vi "Command v1.3.vi"() -> ()   [LabVIEW 2019]
uses:
  <vilib>/ptbypt/NI_PtbyPt.lvlib
panel:
  in  "FU BUTTON FEEDBACK":dbl[](array[numeric])
  out "Array - Numeric":dbl[](array[numeric])
  out "PH LED 6":bool=TRUE
  in  "PH CHECK 6":bool
  out "PH IND 6":bool=TRUE
  in  "CYCLE OX VENT BUTTON":bool
  in  "CYCLE FUEL VENT BUTTON":bool
  in  "DATA INPUT":dbl[](array[numeric])
  in  "INDICATOR INPUT":dbl[](array[numeric])
  out "PH LED 5":bool=TRUE
  out "PH LED 4":bool=TRUE
  out "PH LED 3":bool=TRUE
  out "PH LED 2":bool=TRUE
  out "PH LED 1":bool=TRUE
  in  "PH CHECK 1":bool
  in  "PH CHECK 2":bool
  in  "PH CHECK 3":bool
  in  "PH CHECK 4":bool
  in  "PH CHECK 5":bool
  out "PH IND 5":bool=TRUE
  out "PH IND 4":bool=TRUE
  out "PH IND 3":bool=TRUE
  out "PH IND 2":bool=TRUE
  out "PH IND 1":bool=TRUE
  out "IGN INSERTED BUTTON LED":bool
  in  "IGNITOR IN BUTTON":bool
  in  "MISC BUTTON":bool
  in  "WATER SUP BUTTON":bool
  out "ENGINE TEMP GNG":bool=TRUE
  out "ENGINE PRESS GNG":bool=TRUE
  out "IGNITOR GNG":bool=TRUE
  out "STARTUP GNG":bool=TRUE
  out "SUB PANELS GNG":bool=TRUE
  out "SUB PANEL OX GNG NUM":dbl
  out "SUB PANEL OX GNG LED":bool=TRUE
  out "SUB PANEL FU GNG NUM":dbl
  out "SUB PANEL FU GNG LED":bool=TRUE
  out "VALVE STATES GNG":bool=TRUE
  out "VAVLES ST OX GNG NUM":dbl
  out "VALVE ST OX GNG LED":bool=TRUE
  out "VALVE ST FU GNG NUM":dbl
  out "VALVE ST FU GNG LED":bool=TRUE
  out "PURGE GNG":bool=TRUE
  out "PURGE GNG NUM":dbl
  out "PURGE GNG LED":bool=TRUE
  out "WATER SUP GNG":bool=TRUE
  out "WATER SUP GNG NUM":dbl
  out "WATER SUP GNG LED":bool=TRUE
  out "PRESS VALVES GNG":bool=TRUE
  out "PRESS VALVE OX GNG NUM":dbl
  out "PRESS VALVE OX GNG LED":bool=TRUE
  out "PRESS VALVE FU GNG NUM":dbl
  out "PRESS VALVE FU GNG LED":bool=TRUE
  out "OFFICE GNG":bool=TRUE
  out "RECORD GNG":bool=TRUE
  out "OFFICE GNG NUM":dbl
  out "OFFICE GNG LED":bool=TRUE
  out "RECORD GNG NUM":dbl
  out "RECORD GNG LED":bool=TRUE
  in  "DISABLE BUTTON":bool
  in  "PURGE (1 SEC) BUTTON":bool
  in  "PURGE (2 SEC) BUTTON":bool
  out "TANK PRESS OX METER":dbl(knob) scale=0.0..1600.0
  out "REG PRESS OX METER":dbl(knob) scale=0.0..1600.0
  out "TANK PRESS FU METER":dbl(knob) scale=0.0..1600.0
  out "REG PRESS FU METER":dbl(knob) scale=0.0..1600.0
  in  "RESET":bool
  in  "STOP":bool
  out "ARM GNG":bool=TRUE
  out "IGN IN GNG":bool=TRUE
  out "INJ TEMP GNG":bool=TRUE
  out "CAM GNG":bool=TRUE
  out "PRESS BOTTLE GNG":bool=TRUE
  out "CHILL GNG":bool=TRUE
  out "SYS CYCLE GNG":bool=TRUE
  out "FILL VALVES GNG":bool=TRUE
  out "TANK LEVEL GNG":bool=TRUE
  out "VENT CYCLE GNG":bool=TRUE
  out "ISO VALVE GNG":bool=TRUE
  out "TANK PRESS GNG":bool=TRUE
  out "REG PRESS GNG":bool=TRUE
  out "RELIEF GNG":bool=TRUE
  out "NANNY GNG":bool=TRUE
  out "INJ TEMP GNG NUM":dbl
  out "INJ TEMP GNG LED":bool=TRUE
  out "FILL VALVE OX GNG NUM":dbl
  out "FILL VALVE OX GNG LED":bool=TRUE
  out "ARMED GNG NUM":dbl
  out "ARMED GNG LED":bool=TRUE
  out "TANK LEVEL OX GNG NUM":dbl
  out "TANK LEVEL OX GNG LED":bool=TRUE
  out "VENT CYCLE OX GNG NUM":dbl
  out "VENT CYCLE OX GNG LED":bool=TRUE
  out "PRESS BOTTLE GNG NUM":dbl
  out "PRESS BOTTLE GNG LED":bool=TRUE
  out "ISO VALVE OX GNG NUM":dbl
  out "ISO VALVE OX GNG LED":bool=TRUE
  out "TANK PRESS OX GNG NUM":dbl
  out "TANK PRESS OX GNG LED":bool=TRUE
  out "REG PRESS OX GNG NUM":dbl
  out "REG PRESS OX GNG LED":bool=TRUE
  out "RELIEF OX GNG NUM":dbl
  out "RELIEF OX GNG LED":bool=TRUE
  out "VALVE CYCLE GNG NUM":dbl
  out "SYS CYCLE GNG LED":bool=TRUE
  out "CAM GNG NUM":dbl
  out "CAM GNG LED":bool=TRUE
  out "IGN IN GNG NUM":dbl
  out "IGN IN GNG LED":bool=TRUE
  out "FILL VALVE FU GNG NUM":dbl
  out "FILL VALVE FU GNG LED":bool=TRUE
  out "TANK LEVEL FU GNG NUM":dbl
  out "TANK LEVEL FU GNG LED":bool=TRUE
  out "VENT CYCLE FU GNG NUM":dbl
  out "VENT CYCLE FU GNG LED":bool=TRUE
  out "CHILL GNG NUM":dbl
  out "CHILL GNG LED":bool=TRUE
  out "ISO VALVE FU GNG NUM":dbl
  out "ISO VALVE FU GNG LED":bool=TRUE
  out "TANK PRESS FU GNG NUM":dbl
  out "TANK PRESS FU GNG LED":bool=TRUE
  out "REG PRESS FU GNG NUM":dbl
  out "REG PRESS FU GNG LED":bool=TRUE
  out "RELIEF FU GNG NUM":dbl
  out "RELIEF FU GNG LED":bool=TRUE
  out "NANNY GNG NUM":dbl
  out "NANNY GNG LED":bool=TRUE
  in  "STARTUP BUTTON":bool
  out "PT COMBUSTION CHAMBER":dbl
  in  "SYS GNG BUTTON":bool=TRUE
  out "REC DATA BUTTON LED":bool
  in  "RECORD DATA BUTTON":bool
  out "CC TEMP 3":dbl(slide) scale=-150.0..500.0
  out "CC TEMP 2":dbl(slide) scale=-150.0..500.0
  out "CC TEMP 1":dbl(slide) scale=-150.0..500.0
  out "OX CHILL TEMP":dbl(slide) scale=-200.0..75.0
  out "OFFICE GNG BUTTON LED":bool
  in  "OFFICE GNG BUTTON":bool
  out "CAM GNG BUTTON LED":bool
  in  "CAM GNG BUTTON":bool
  out "OX TANK TEMP 4":dbl(slide) scale=-200.0..75.0
  out "OX TANK TEMP 3":dbl(slide) scale=-200.0..75.0
  out "OX TANK TEMP 5":dbl(slide) scale=-200.0..75.0
  out "OX TANK TEMP 1":dbl(slide) scale=-200.0..75.0
  out "ARMED PANEL LED":bool
  out "IGN INSERTED PANEL LED":bool
  out "NANNY PAN LED":bool
  out "FUEL VENT CYCLE BUTTON LED":bool
  out "OX VENT CYCLE BUTTON LED":bool
  in  "VALVE SEQ BUTTON":bool
  in  "FIRE BUTTON":bool
  out "PT FU MAIN VALVE":dbl
  out "PT FU VENTURI":dbl
  out "PT OX MAIN VALVE":dbl
  out "PT OX VENTURI":dbl
  out "FUEL TANK RELIEF TEMP":dbl(slide) scale=-200.0..75.0
  out "FUELTANK TEMP":dbl(slide) scale=-200.0..75.0
  out "OX TANK RELIEF TEMP":dbl(slide) scale=-200.0..75.0
  out "OX LINE RELIEF TEMP":dbl(slide) scale=-200.0..75.0
  in  "ABORT BUTTON":bool
  in  "COMMAND GNG BUTTON":bool=TRUE
  out "OX SUB PANEL GNG MAIN":bool=TRUE
  out "FU SUB PANEL GNG MAIN":bool=TRUE
  out "SYS STATE FU STRING":string
  out "SYS STATE OX STRING":string
  out "FUEL TANK LEVEL (%) 2":dbl(slide) scale=0.0..100.0
  in  "ABV-OX-250 (OX FILL)":bool
  out "ABV-OX-250 LED":bool=TRUE
  in  "ABV-OX-240 (OX CHILL)":bool
  out "ABV-OX-240 LED":bool=TRUE
  in  "ABV-OX-230 (OX MAIN)":bool
  out "ABV-OX-230 LED":bool=TRUE
  in  "ABV-OX-220 (OX ISO)":bool
  out "ABV-OX-220 LED":bool=TRUE
  in  "ABV-OX-210 (OX VENT)":bool
  out "ABV-OX-210 LED":bool=TRUE
  in  "ABV-PR-110 (OX PRESS)":bool
  out "ABV-PR-110 LED":bool=TRUE
  in  "NANNY MODE BUTTON":bool
  out "PT PRESSURANT":dbl(slide) scale=0.0..10.0
  out "SYS STATE MAIN STRING":string
  out "FUEL TANK LEVEL (%)":dbl(slide) scale=0.0..100.0
  in  "FUEL FILL BUTTON":bool
  out "FUEL FILL LED":bool=TRUE
  in  "ABV-FU-340 (FUEL PURGE)":bool
  out "ABV-FU-340 LED":bool=TRUE
  in  "ABV-FU-330 (FUEL MAIN)":bool
  out "ABV-FU-330 LED":bool=TRUE
  in  "ABV-FU-320 (FUEL ISO)":bool
  out "ABV-FU-320 LED":bool=TRUE
  in  "ABV-FU-310 (FUEL VENT)":bool
  out "ABV-FU-310 LED":bool=TRUE
  in  "ABV-PR-120 (FUEL PRESS)":bool
  out "ABV-PR-120 LED":bool=TRUE
  # "Ox CONTROL"
  # "FUEL CONTROL"
  # "NANNY"
  # "IGNITOR \nINSERTED"
  # "ARMED"
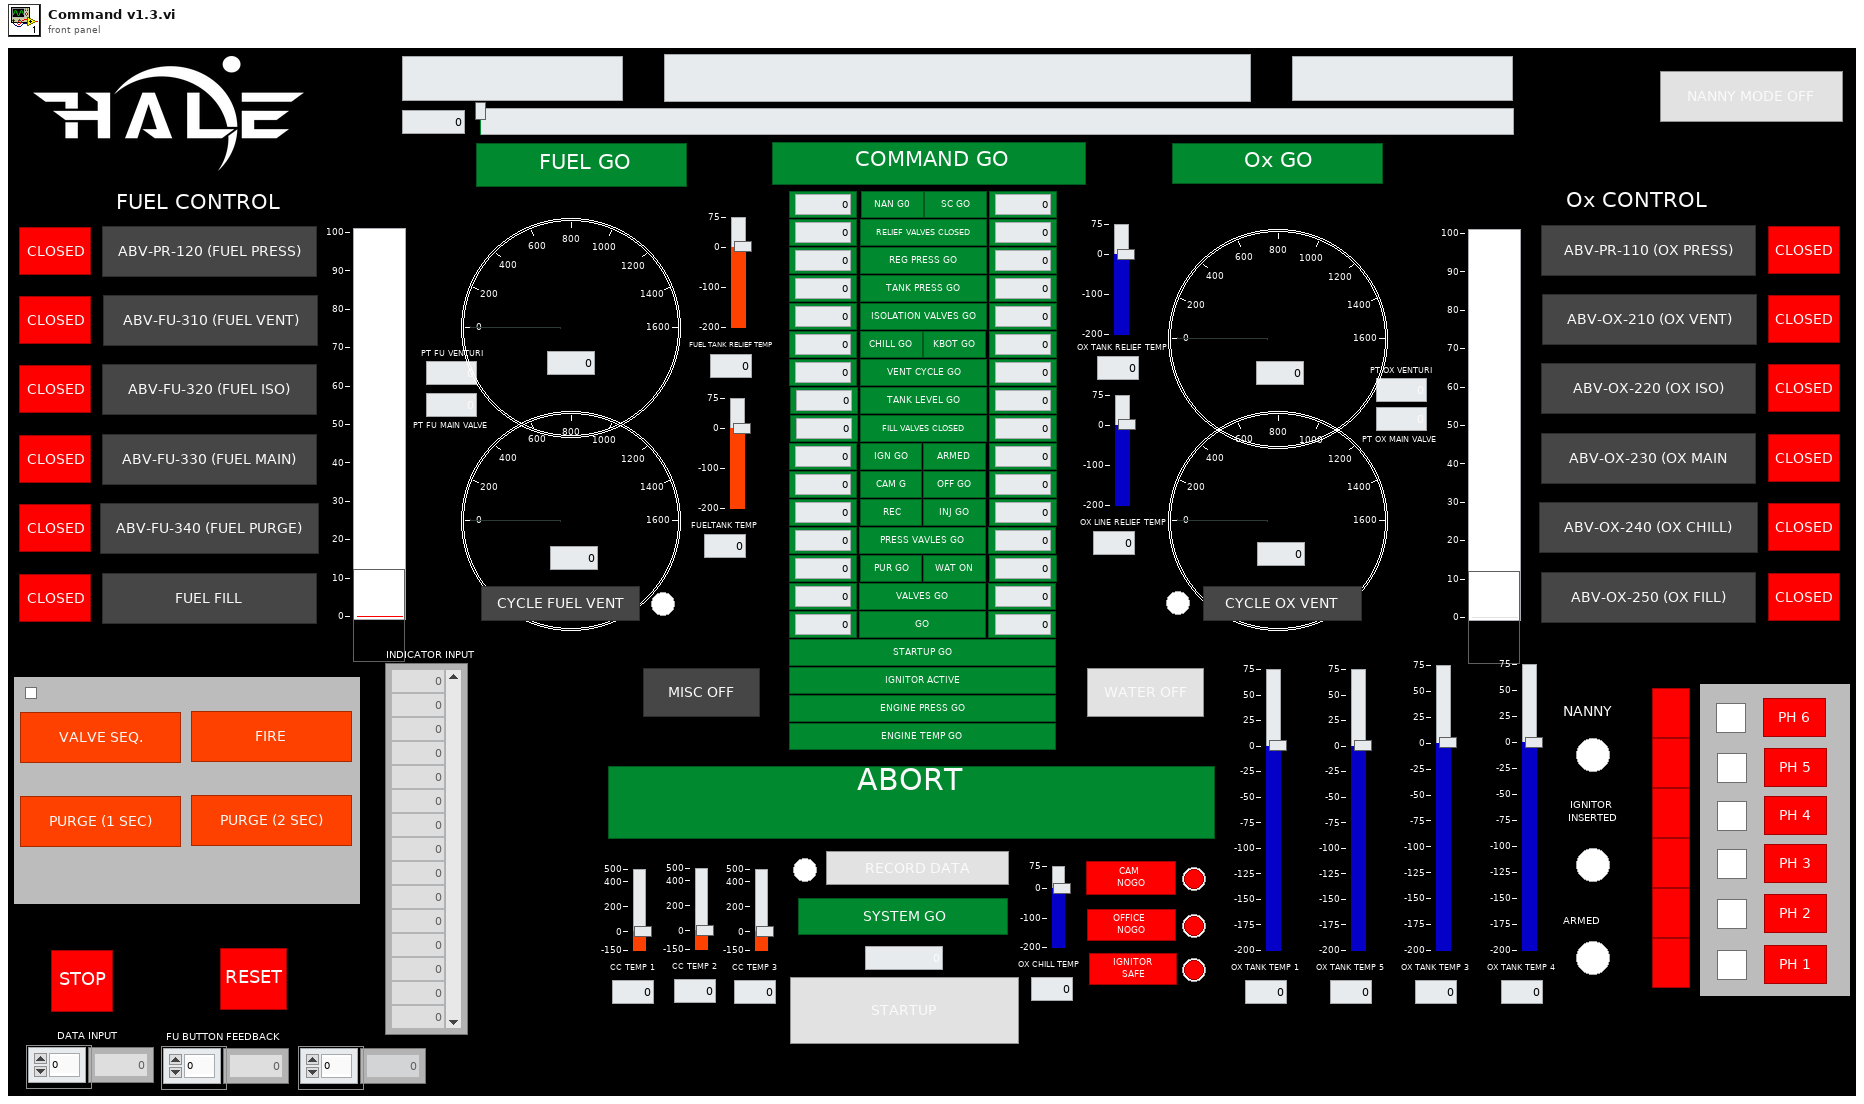
[diagram p1: front panel]
types:
  T1 = enum8{"Enabled", "Disabled", "Disabled and Grayed Out"}
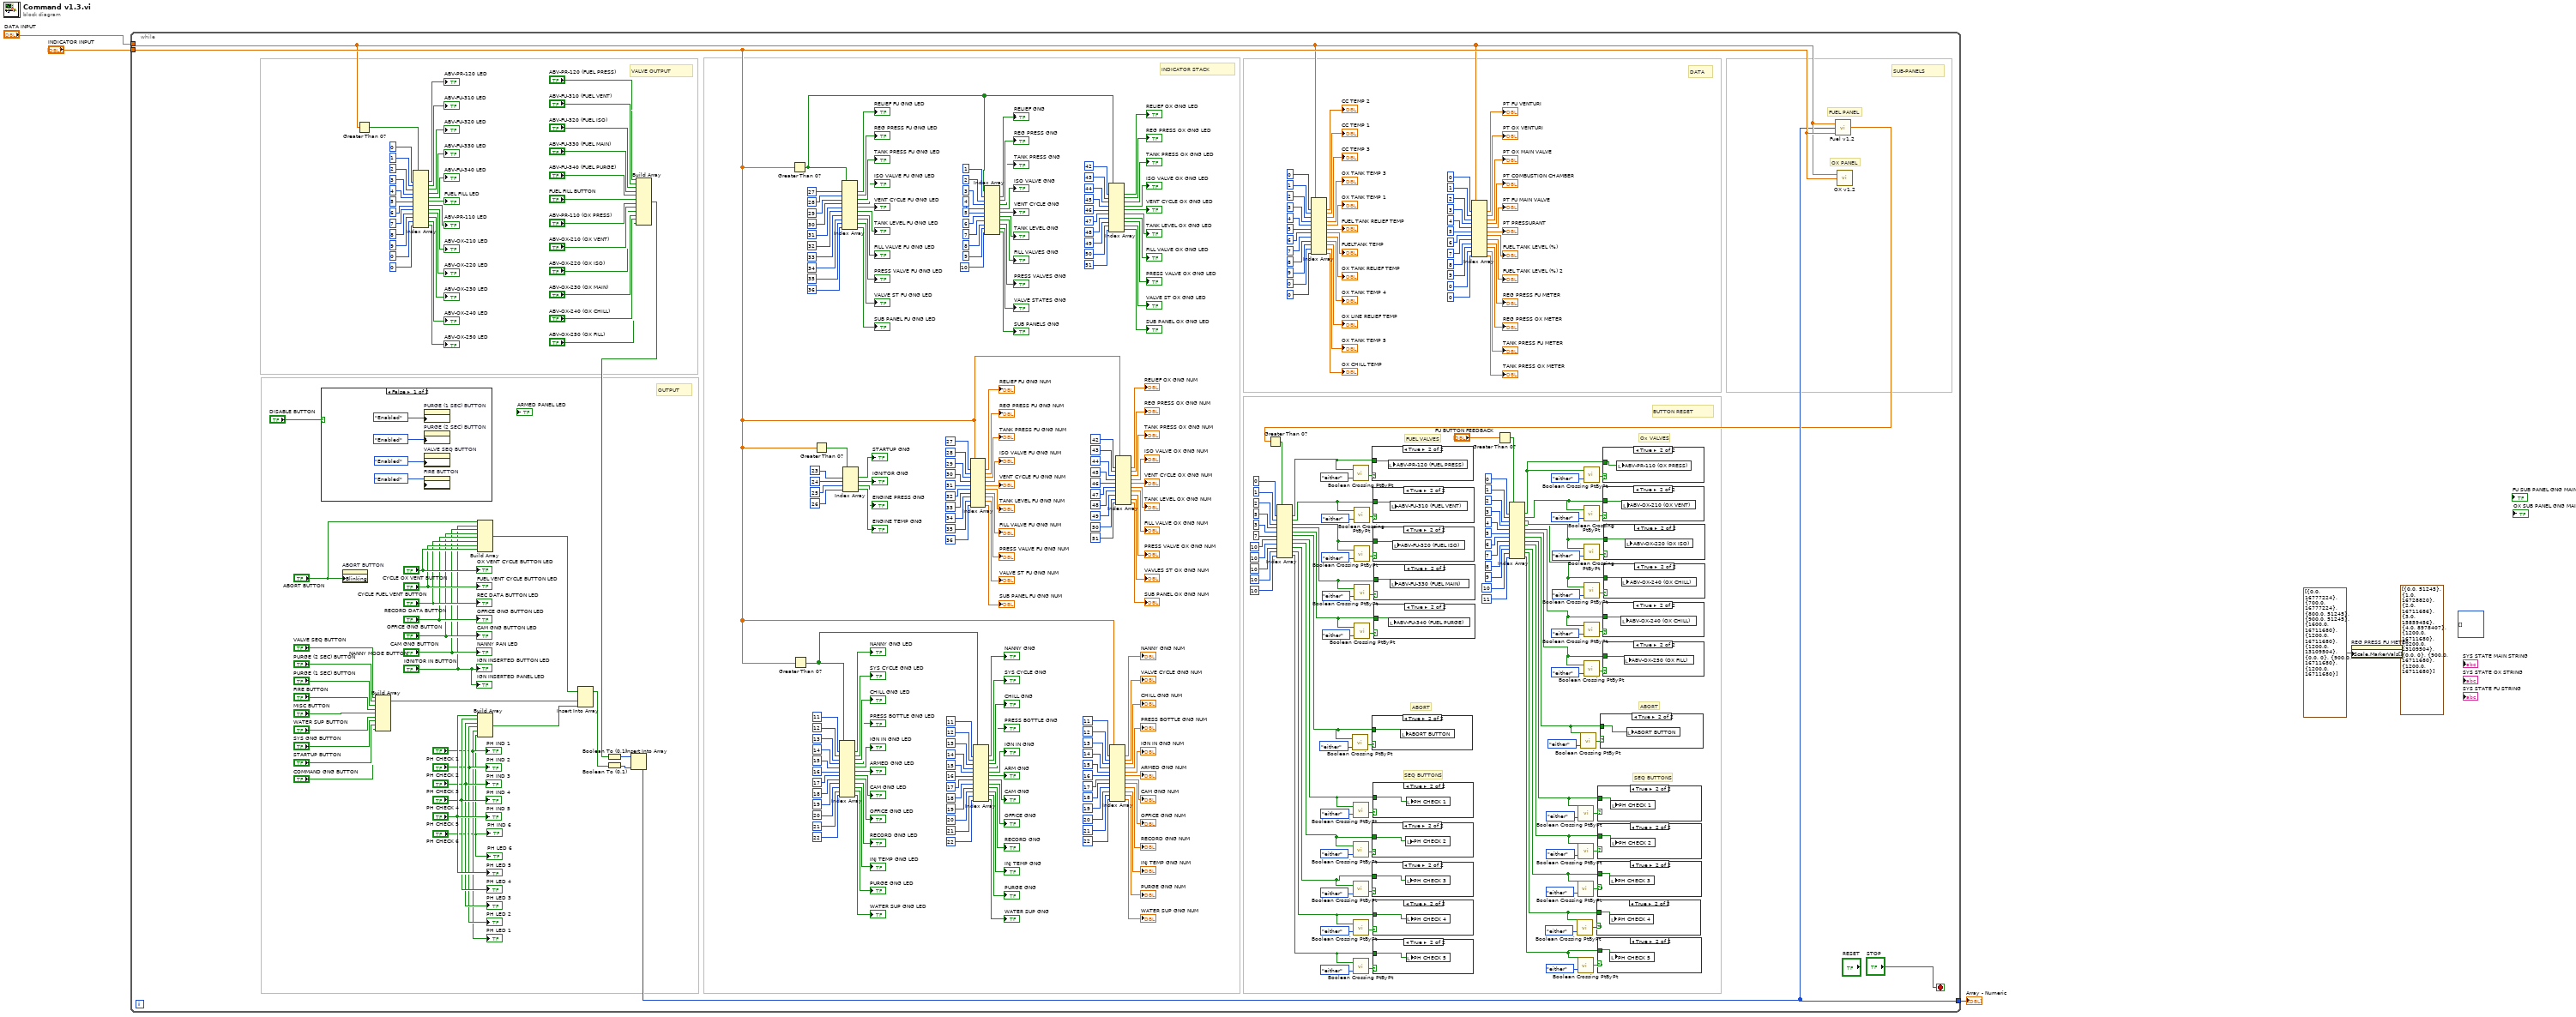
[diagram p0: block diagram]
diagram:
  (unwired) u32[] [] ("Scale.Marker Values[]")
  (unwired) cluster{dbl, u32}[] [{0.0, 51245}, {1.0, 16728820}, {2.0, 16711686}, {3.0, 15859456}, {4.0, 8978407}, {1200.0, 16711680}, {1200.0, 13109504}, {0.0, 0}, {900.0, 16711680}, {1200.0, 16711680}] ("Scale.Marker Values[]")
  n1 = while {
    tunnel: "INDICATOR INPUT" -> [w16]
    tunnel: "DATA INPUT" -> [w15]
    tunnel: [w6] -> w1
    stop <- "STOP" stop-if-true
    # "SUB-PANELS"
    # "FUEL PANEL"
    # "OX PANEL"
    # "SEQ BUTTONS"
    # "ABORT"
    # "SEQ BUTTONS"
    # "ABORT"
    # "FUEL VALVES"
    # "Ox VALVES"
    # "BUTTON RESET"
    # "DATA"
    # "INDICATOR STACK"
    # "VALVE OUTPUT"
    # "OUTPUT"
    n2 = case shown="False" "DISABLE BUTTON" {
      frame False {
        n3 = property on="PURGE (1 SEC) BUTTON" class="Bool (strict)"("DisabledEnum"=T1."Enabled" ("Disabled")) -> ()  [unwired: 2 in, 2 out]
        n4 = property on="PURGE (2 SEC) BUTTON" class="Bool (strict)"("DisabledEnum"=T1."Enabled" ("Disabled")) -> ()  [unwired: 2 in, 2 out]
        n5 = property on="VALVE SEQ BUTTON" class="Bool (strict)"("DisabledEnum"=T1."Enabled" ("Disabled")) -> ()  [unwired: 2 in, 2 out]
        n6 = property on="FIRE BUTTON" class="Bool (strict)"("DisabledEnum"=T1."Enabled" ("Disabled")) -> ()  [unwired: 2 in, 2 out]
      }
      frame True {
        n7 = property on="VALVE SEQ BUTTON" class="Bool (strict)"("DisabledEnum"=T1."Disabled and Grayed Out" ("Disabled")) -> ()  [unwired: 2 in, 2 out]
        n8 = property on="PURGE (2 SEC) BUTTON" class="Bool (strict)"("DisabledEnum"=T1."Disabled and Grayed Out" ("Disabled")) -> ()  [unwired: 2 in, 2 out]
        n9 = property on="FIRE BUTTON" class="Bool (strict)"("DisabledEnum"=T1."Disabled and Grayed Out" ("Disabled")) -> ()  [unwired: 2 in, 2 out]
        n10 = property on="PURGE (1 SEC) BUTTON" class="Bool (strict)"("DisabledEnum"=T1."Disabled and Grayed Out" ("Disabled")) -> ()  [unwired: 2 in, 2 out]
      }
    }
    n11 = property on="ABORT BUTTON" class="Bool (strict)"("Blinking"="ABORT BUTTON") -> ()  [unwired: 2 in, 2 out]
    n12 = Greater Than 0?(x=w15) -> (x > 0?=w148:bool[])
    n13 = Build Array("VALVE SEQ BUTTON", "PURGE (2 SEC) BUTTON", "PURGE (1 SEC) BUTTON", "FIRE BUTTON", "MISC BUTTON", "WATER SUP BUTTON", "SYS GNG BUTTON", "STARTUP BUTTON", "COMMAND GNG BUTTON") -> (w11:bool[])
    n14 = Index Array(array=w148, index #1=0 ("index"), index #2=1 ("index"), index #3=2 ("index"), index #4=3 ("index"), index #5=4 ("index"), index #6=5 ("index"), index #7=6 ("index"), index #8=7 ("index"), index #9=8 ("index"), index #10=9 ("index"), index #11=0 ("index"), index #12=0 ("index")) -> (element #1=→"ABV-PR-120 LED":bool, element #2=→"ABV-FU-310 LED":bool, element #3=→"ABV-FU-320 LED":bool, element #4=→"ABV-FU-330 LED":bool, element #5=→"ABV-FU-340 LED":bool, element #6=→"FUEL FILL LED":bool, element #7=→"ABV-PR-110 LED":bool, element #8=→"ABV-OX-210 LED":bool, element #9=→"ABV-OX-220 LED":bool, element #10=→"ABV-OX-230 LED":bool, element #11=→"ABV-OX-240 LED":bool, element #12=→"ABV-OX-250 LED":bool)
    n15 = Build Array("ABORT BUTTON", "IGNITOR IN BUTTON", "NANNY MODE BUTTON", "CAM GNG BUTTON", "OFFICE GNG BUTTON", "RECORD DATA BUTTON", "CYCLE FUEL VENT BUTTON", "CYCLE OX VENT BUTTON") -> (w13:bool[])
    n16 = Build Array("PH CHECK 5", "PH CHECK 4", "PH CHECK 3", "PH CHECK 2", "PH CHECK 1", "PH CHECK 6") -> (w12:bool[])
    n17 = Insert Into Array(array=w13, new element #1=w11, new element #2=w12) -> (w10:bool[])  [unwired: 1 in]
    n18 = Boolean To (0,1)(Boolean=w10) -> (0, 1=w8:i16[])
    n19 = Build Array("ABV-PR-120 (FUEL PRESS)", "ABV-FU-310 (FUEL VENT)", "ABV-FU-320 (FUEL ISO)", "ABV-FU-330 (FUEL MAIN)", "ABV-FU-340 (FUEL PURGE)", "FUEL FILL BUTTON", "ABV-PR-110 (OX PRESS)", "ABV-OX-210 (OX VENT)", "ABV-OX-220 (OX ISO)", "ABV-OX-230 (OX MAIN)", "ABV-OX-240 (OX CHILL)", "ABV-OX-250 (OX FILL)") -> (w14:bool[])
    n20 = Boolean To (0,1)(Boolean=w14) -> (0, 1=w9:i16[])
    n21 = Insert Into Array(array=w9, new element=w8) -> (w6:i16[])  [unwired: 1 in]
    n22 = Greater Than 0?(x=w16) -> (x > 0?=w127:bool[])
    n23 = Greater Than 0?(x=w16) -> (x > 0?=w275:bool[])
    n24 = Greater Than 0?(x=w16) -> (x > 0?=w118:bool[])
    n25 = Index Array(array=w275, index #1=11 ("index"), index #2=12 ("index"), index #3=13 ("index"), index #4=14 ("index"), index #5=15 ("index"), index #6=16 ("index"), index #7=17 ("index"), index #8=18 ("index"), index #9=19 ("index"), index #10=20 ("index"), index #11=21 ("index"), index #12=22 ("index")) -> (element #1=→"NANNY GNG LED":bool, element #2=→"SYS CYCLE GNG LED":bool, element #3=→"CHILL GNG LED":bool, element #4=→"PRESS BOTTLE GNG LED":bool, element #5=→"IGN IN GNG LED":bool, element #6=→"ARMED GNG LED":bool, element #7=→"CAM GNG LED":bool, element #8=→"OFFICE GNG LED":bool, element #9=→"RECORD GNG LED":bool, element #10=→"INJ TEMP GNG LED":bool, element #11=→"PURGE GNG LED":bool, element #12=→"WATER SUP GNG LED":bool)
    n26 = Index Array(array=w127, index #1=27 ("index"), index #2=28 ("index"), index #3=29 ("index"), index #4=30 ("index"), index #5=31 ("index"), index #6=32 ("index"), index #7=33 ("index"), index #8=34 ("index"), index #9=35 ("index"), index #10=36 ("index")) -> (element #1=→"RELIEF FU GNG LED":bool, element #2=→"REG PRESS FU GNG LED":bool, element #3=→"TANK PRESS FU GNG LED":bool, element #4=→"ISO VALVE FU GNG LED":bool, element #5=→"VENT CYCLE FU GNG LED":bool, element #6=→"TANK LEVEL FU GNG LED":bool, element #7=→"FILL VALVE FU GNG LED":bool, element #8=→"PRESS VALVE FU GNG LED":bool, element #9=→"VALVE ST FU GNG LED":bool, element #10=→"SUB PANEL FU GNG LED":bool)
    n27 = Index Array(array=w118, index #1=23 ("index"), index #2=24 ("index"), index #3=25 ("index"), index #4=26 ("index")) -> (element #1=→"STARTUP GNG":bool, element #2=→"IGNITOR GNG":bool, element #3=→"ENGINE PRESS GNG":bool, element #4=→"ENGINE TEMP GNG":bool)
    n28 = Index Array(array=w16, index #1=27 ("index"), index #2=28 ("index"), index #3=29 ("index"), index #4=30 ("index"), index #5=31 ("index"), index #6=32 ("index"), index #7=33 ("index"), index #8=34 ("index"), index #9=35 ("index"), index #10=36 ("index")) -> (element #1=→"RELIEF FU GNG NUM":dbl, element #2=→"REG PRESS FU GNG NUM":dbl, element #3=→"TANK PRESS FU GNG NUM":dbl, element #4=→"ISO VALVE FU GNG NUM":dbl, element #5=→"VENT CYCLE FU GNG NUM":dbl, element #6=→"TANK LEVEL FU GNG NUM":dbl, element #7=→"FILL VALVE FU GNG NUM":dbl, element #8=→"PRESS VALVE FU GNG NUM":dbl, element #9=→"VALVE ST FU GNG NUM":dbl, element #10=→"SUB PANEL FU GNG NUM":dbl)
    n29 = Index Array(array=w275, index #1=11 ("index"), index #2=12 ("index"), index #3=13 ("index"), index #4=14 ("index"), index #5=15 ("index"), index #6=16 ("index"), index #7=17 ("index"), index #8=18 ("index"), index #9=19 ("index"), index #10=20 ("index"), index #11=21 ("index"), index #12=22 ("index")) -> (element #1=→"NANNY GNG":bool, element #2=→"SYS CYCLE GNG":bool, element #3=→"CHILL GNG":bool, element #4=→"PRESS BOTTLE GNG":bool, element #5=→"IGN IN GNG":bool, element #6=→"ARM GNG":bool, element #7=→"CAM GNG":bool, element #8=→"OFFICE GNG":bool, element #9=→"RECORD GNG":bool, element #10=→"INJ TEMP GNG":bool, element #11=→"PURGE GNG":bool, element #12=→"WATER SUP GNG":bool)
    n30 = Index Array(array=w127, index #1=1 ("index"), index #2=2 ("index"), index #3=3 ("index"), index #4=4 ("index"), index #5=5 ("index"), index #6=6 ("index"), index #7=7 ("index"), index #8=8 ("index"), index #9=9 ("index"), index #10=10 ("index")) -> (element #1=→"RELIEF GNG":bool, element #2=→"REG PRESS GNG":bool, element #3=→"TANK PRESS GNG":bool, element #4=→"ISO VALVE GNG":bool, element #5=→"VENT CYCLE GNG":bool, element #6=→"TANK LEVEL GNG":bool, element #7=→"FILL VALVES GNG":bool, element #8=→"PRESS VALVES GNG":bool, element #9=→"VALVE STATES GNG":bool, element #10=→"SUB PANELS GNG":bool)
    n31 = Index Array(array=w127, index #1=42 ("index"), index #2=43 ("index"), index #3=44 ("index"), index #4=45 ("index"), index #5=46 ("index"), index #6=47 ("index"), index #7=48 ("index"), index #8=49 ("index"), index #9=50 ("index"), index #10=51 ("index")) -> (element #1=→"RELIEF OX GNG LED":bool, element #2=→"REG PRESS OX GNG LED":bool, element #3=→"TANK PRESS OX GNG LED":bool, element #4=→"ISO VALVE OX GNG LED":bool, element #5=→"VENT CYCLE OX GNG LED":bool, element #6=→"TANK LEVEL OX GNG LED":bool, element #7=→"FILL VALVE OX GNG LED":bool, element #8=→"PRESS VALVE OX GNG LED":bool, element #9=→"VALVE ST OX GNG LED":bool, element #10=→"SUB PANEL OX GNG LED":bool)
    n32 = Index Array(array=w16, index #1=11 ("index"), index #2=12 ("index"), index #3=13 ("index"), index #4=14 ("index"), index #5=15 ("index"), index #6=16 ("index"), index #7=17 ("index"), index #8=18 ("index"), index #9=19 ("index"), index #10=20 ("index"), index #11=21 ("index"), index #12=22 ("index")) -> (element #1=→"NANNY GNG NUM":dbl, element #2=→"VALVE CYCLE GNG NUM":dbl, element #3=→"CHILL GNG NUM":dbl, element #4=→"PRESS BOTTLE GNG NUM":dbl, element #5=→"IGN IN GNG NUM":dbl, element #6=→"ARMED GNG NUM":dbl, element #7=→"CAM GNG NUM":dbl, element #8=→"OFFICE GNG NUM":dbl, element #9=→"RECORD GNG NUM":dbl, element #10=→"INJ TEMP GNG NUM":dbl, element #11=→"PURGE GNG NUM":dbl, element #12=→"WATER SUP GNG NUM":dbl)
    n33 = Index Array(array=w16, index #1=42 ("index"), index #2=43 ("index"), index #3=44 ("index"), index #4=45 ("index"), index #5=46 ("index"), index #6=47 ("index"), index #7=48 ("index"), index #8=49 ("index"), index #9=50 ("index"), index #10=51 ("index")) -> (element #1=→"RELIEF OX GNG NUM":dbl, element #2=→"REG PRESS OX GNG NUM":dbl, element #3=→"TANK PRESS OX GNG NUM":dbl, element #4=→"ISO VALVE OX GNG NUM":dbl, element #5=→"VENT CYCLE OX GNG NUM":dbl, element #6=→"TANK LEVEL OX GNG NUM":dbl, element #7=→"FILL VALVE OX GNG NUM":dbl, element #8=→"PRESS VALVE OX GNG NUM":dbl, element #9=→"VAVLES ST OX GNG NUM":dbl, element #10=→"SUB PANEL OX GNG NUM":dbl)
    n34 = Index Array(array=w15, index #1=0 ("index"), index #2=1 ("index"), index #3=2 ("index"), index #4=3 ("index"), index #5=4 ("index"), index #6=5 ("index"), index #7=6 ("index"), index #8=7 ("index"), index #9=8 ("index"), index #10=9 ("index"), index #11=0 ("index"), index #12=0 ("index")) -> (element #1=→"CC TEMP 2":dbl, element #2=→"CC TEMP 1":dbl, element #3=→"CC TEMP 3":dbl, element #4=→"OX TANK TEMP 3":dbl, element #5=→"OX TANK TEMP 1":dbl, element #6=→"FUEL TANK RELIEF TEMP":dbl, element #7=→"FUELTANK TEMP":dbl, element #8=→"OX TANK RELIEF TEMP":dbl, element #9=→"OX TANK TEMP 4":dbl, element #10=→"OX LINE RELIEF TEMP":dbl, element #11=→"OX TANK TEMP 5":dbl, element #12=→"OX CHILL TEMP":dbl)
    n35 = Index Array(array=w15, index #1=0 ("index"), index #2=1 ("index"), index #3=2 ("index"), index #4=3 ("index"), index #5=4 ("index"), index #6=5 ("index"), index #7=6 ("index"), index #8=7 ("index"), index #9=8 ("index"), index #10=9 ("index"), index #11=0 ("index"), index #12=0 ("index")) -> (element #1=→"PT FU VENTURI":dbl, element #2=→"PT OX VENTURI":dbl, element #3=→"PT OX MAIN VALVE":dbl, element #4=→"PT COMBUSTION CHAMBER":dbl, element #5=→"PT FU MAIN VALVE":dbl, element #6=→"PT PRESSURANT":dbl, element #7=→"FUEL TANK LEVEL (%)":dbl, element #8=→"FUEL TANK LEVEL (%) 2":dbl, element #9=→"REG PRESS FU METER":dbl, element #10=→"REG PRESS OX METER":dbl, element #11=→"TANK PRESS FU METER":dbl, element #12=→"TANK PRESS OX METER":dbl)
    n36 = Greater Than 0?(x="FU BUTTON FEEDBACK") -> (x > 0?=w43:bool[])
    n37 = Index Array(array=w43, index #1=0 ("index"), index #2=1 ("index"), index #3=2 ("index"), index #4=3 ("index"), index #5=4 ("index"), index #6=5 ("index"), index #7=6 ("index"), index #8=7 ("index"), index #9=8 ("index"), index #10=9 ("index"), index #11=10 ("index"), index #12=11 ("index")) -> (element #1=w41:bool, element #2=w48:bool, element #3=w47:bool, element #4=w46:bool, element #5=w45:bool, element #6=w44:bool, element #7=w28:bool, element #8=w27:bool, element #9=w26:bool, element #10=w25:bool, element #11=w24:bool, element #12=w23:bool)
    n38 = call <vilib>:"Boolean Crossing PtByPt.vi"("direction"=enum16{"either", "false-true", "true-false"}."either", "input"=w24) -> ("crossing"=w36:bool)  [unwired: 1 in]
    n39 = call <vilib>:"Boolean Crossing PtByPt.vi"("direction"=enum16{"either", "false-true", "true-false"}."either", "input"=w25) -> ("crossing"=w38:bool)  [unwired: 1 in]
    n40 = call <vilib>:"Boolean Crossing PtByPt.vi"("direction"=enum16{"either", "false-true", "true-false"}."either", "input"=w23) -> ("crossing"=w34:bool)  [unwired: 1 in]
    n41 = call <vilib>:"Boolean Crossing PtByPt.vi"("direction"=enum16{"either", "false-true", "true-false"}."either", "input"=w27) -> ("crossing"=w30:bool)  [unwired: 1 in]
    n42 = call <vilib>:"Boolean Crossing PtByPt.vi"("direction"=enum16{"either", "false-true", "true-false"}."either", "input"=w26) -> ("crossing"=w32:bool)  [unwired: 1 in]
    n43 = call <vilib>:"Boolean Crossing PtByPt.vi"("direction"=enum16{"either", "false-true", "true-false"}."either", "input"=w28) -> ("crossing"=w40:bool)  [unwired: 1 in]
    n44 = call <vilib>:"Boolean Crossing PtByPt.vi"("direction"=enum16{"either", "false-true", "true-false"}."either", "input"=w41) -> ("crossing"=w83:bool)  [unwired: 1 in]
    n45 = call <vilib>:"Boolean Crossing PtByPt.vi"("direction"=enum16{"either", "false-true", "true-false"}."either", "input"=w48) -> ("crossing"=w81:bool)  [unwired: 1 in]
    n46 = call <vilib>:"Boolean Crossing PtByPt.vi"("direction"=enum16{"either", "false-true", "true-false"}."either", "input"=w45) -> ("crossing"=w75:bool)  [unwired: 1 in]
    n47 = call <vilib>:"Boolean Crossing PtByPt.vi"("direction"=enum16{"either", "false-true", "true-false"}."either", "input"=w44) -> ("crossing"=w73:bool)  [unwired: 1 in]
    n48 = call <vilib>:"Boolean Crossing PtByPt.vi"("direction"=enum16{"either", "false-true", "true-false"}."either", "input"=w47) -> ("crossing"=w79:bool)  [unwired: 1 in]
    n49 = call <vilib>:"Boolean Crossing PtByPt.vi"("direction"=enum16{"either", "false-true", "true-false"}."either", "input"=w46) -> ("crossing"=w77:bool)  [unwired: 1 in]
    n50 = case shown="True" w36 {
      tunnel: w24 -> [_ w407]
      frame False {
      }
      frame True {
        n51 = local write "PH CHECK 4"(w407) -> ()
      }
    }
    n52 = case shown="True" w38 {
      tunnel: w25 -> [_ w408]
      frame False {
      }
      frame True {
        n53 = local write "PH CHECK 3"(w408) -> ()
      }
    }
    n54 = case shown="True" w34 {
      tunnel: w23 -> [_ w406]
      frame False {
      }
      frame True {
        n55 = local write "PH CHECK 5"(w406) -> ()
      }
    }
    n56 = case shown="True" w30 {
      tunnel: w27 -> [_ w404]
      frame False {
      }
      frame True {
        n57 = local write "PH CHECK 1"(w404) -> ()
      }
    }
    n58 = case shown="True" w32 {
      tunnel: w26 -> [_ w405]
      frame False {
      }
      frame True {
        n59 = local write "PH CHECK 2"(w405) -> ()
      }
    }
    n60 = case shown="True" w40 {
      tunnel: w28 -> [_ w409]
      frame False {
      }
      frame True {
        n61 = local write "ABORT BUTTON"(w409) -> ()
      }
    }
    n62 = case shown="True" w83 {
      tunnel: w41 -> [_ w421]
      frame False {
      }
      frame True {
        n63 = local write "ABV-PR-110 (OX PRESS)"(w421) -> ()
      }
    }
    n64 = case shown="True" w81 {
      tunnel: w48 -> [_ w420]
      frame False {
      }
      frame True {
        n65 = local write "ABV-OX-210 (OX VENT)"(w420) -> ()
      }
    }
    n66 = case shown="True" w75 {
      tunnel: w45 -> [_ w417]
      frame False {
      }
      frame True {
        n67 = local write "ABV-OX-240 (OX CHILL)"(w417) -> ()
      }
    }
    n68 = case shown="True" w73 {
      tunnel: w44 -> [_ w416]
      frame False {
      }
      frame True {
        n69 = local write "ABV-OX-250 (OX FILL)"(w416) -> ()
      }
    }
    n70 = case shown="True" w79 {
      tunnel: w47 -> [_ w419]
      frame False {
      }
      frame True {
        n71 = local write "ABV-OX-220 (OX ISO)"(w419) -> ()
      }
    }
    n72 = case shown="True" w77 {
      tunnel: w46 -> [_ w418]
      frame False {
      }
      frame True {
        n73 = local write "ABV-OX-240 (OX CHILL)"(w418) -> ()
      }
    }
    n74 = call "Fuel v1.2.vi"("INDICATOR INPUT"=w16, "BUTTON INPUT"=w6, "DATA INPUT"=w15) -> ("OUTPUT"=w5:dbl[])
    n75 = Greater Than 0?(x=w5) -> (x > 0?=w42:bool[])
    n76 = Index Array(array=w42, index #1=0 ("index"), index #2=1 ("index"), index #3=2 ("index"), index #4=5 ("index"), index #5=3 ("index"), index #6=7 ("index"), index #7=10 ("index"), index #8=10 ("index"), index #9=10 ("index"), index #10=10 ("index"), index #11=10 ("index")) -> (element #1=w59:bool, element #2=w58:bool, element #3=w57:bool, element #4=w56:bool, element #5=w55:bool, element #6=w54:bool, element #7=w53:bool, element #8=w52:bool, element #9=w51:bool, element #10=w50:bool, element #11=w49:bool)
    n77 = call <vilib>:"Boolean Crossing PtByPt.vi"("direction"=enum16{"either", "false-true", "true-false"}."either", "input"=w54) -> ("crossing"=w71:bool)  [unwired: 1 in]
    n78 = call <vilib>:"Boolean Crossing PtByPt.vi"("direction"=enum16{"either", "false-true", "true-false"}."either", "input"=w59) -> ("crossing"=w116:bool)  [unwired: 1 in]
    n79 = call <vilib>:"Boolean Crossing PtByPt.vi"("direction"=enum16{"either", "false-true", "true-false"}."either", "input"=w52) -> ("crossing"=w67:bool)  [unwired: 1 in]
    n80 = call <vilib>:"Boolean Crossing PtByPt.vi"("direction"=enum16{"either", "false-true", "true-false"}."either", "input"=w51) -> ("crossing"=w65:bool)  [unwired: 1 in]
    n81 = call <vilib>:"Boolean Crossing PtByPt.vi"("direction"=enum16{"either", "false-true", "true-false"}."either", "input"=w53) -> ("crossing"=w69:bool)  [unwired: 1 in]
    n82 = call <vilib>:"Boolean Crossing PtByPt.vi"("direction"=enum16{"either", "false-true", "true-false"}."either", "input"=w50) -> ("crossing"=w63:bool)  [unwired: 1 in]
    n83 = call <vilib>:"Boolean Crossing PtByPt.vi"("direction"=enum16{"either", "false-true", "true-false"}."either", "input"=w49) -> ("crossing"=w61:bool)  [unwired: 1 in]
    n84 = call <vilib>:"Boolean Crossing PtByPt.vi"("direction"=enum16{"either", "false-true", "true-false"}."either", "input"=w58) -> ("crossing"=w91:bool)  [unwired: 1 in]
    n85 = call <vilib>:"Boolean Crossing PtByPt.vi"("direction"=enum16{"either", "false-true", "true-false"}."either", "input"=w57) -> ("crossing"=w89:bool)  [unwired: 1 in]
    n86 = call <vilib>:"Boolean Crossing PtByPt.vi"("direction"=enum16{"either", "false-true", "true-false"}."either", "input"=w56) -> ("crossing"=w87:bool)  [unwired: 1 in]
    n87 = call <vilib>:"Boolean Crossing PtByPt.vi"("direction"=enum16{"either", "false-true", "true-false"}."either", "input"=w55) -> ("crossing"=w85:bool)  [unwired: 1 in]
    n88 = case shown="True" w71 {
      tunnel: w54 -> [_ w415]
      frame False {
      }
      frame True {
        n89 = local write "ABORT BUTTON"(w415) -> ()
      }
    }
    n90 = case shown="True" w116 {
      tunnel: w59 -> [_ w426]
      frame False {
      }
      frame True {
        n91 = local write "ABV-PR-120 (FUEL PRESS)"(w426) -> ()
      }
    }
    n92 = case shown="True" w67 {
      tunnel: w52 -> [_ w413]
      frame False {
      }
      frame True {
        n93 = local write "PH CHECK 2"(w413) -> ()
      }
    }
    n94 = case shown="True" w65 {
      tunnel: w51 -> [_ w412]
      frame False {
      }
      frame True {
        n95 = local write "PH CHECK 3"(w412) -> ()
      }
    }
    n96 = case shown="True" w69 {
      tunnel: w53 -> [_ w414]
      frame False {
      }
      frame True {
        n97 = local write "PH CHECK 1"(w414) -> ()
      }
    }
    n98 = case shown="True" w63 {
      tunnel: w50 -> [_ w411]
      frame False {
      }
      frame True {
        n99 = local write "PH CHECK 4"(w411) -> ()
      }
    }
    n100 = case shown="True" w61 {
      tunnel: w49 -> [_ w410]
      frame False {
      }
      frame True {
        n101 = local write "PH CHECK 5"(w410) -> ()
      }
    }
    n102 = case shown="True" w91 {
      tunnel: w58 -> [_ w425]
      frame False {
      }
      frame True {
        n103 = local write "ABV-FU-310 (FUEL VENT)"(w425) -> ()
      }
    }
    n104 = case shown="True" w89 {
      tunnel: w57 -> [_ w424]
      frame False {
      }
      frame True {
        n105 = local write "ABV-FU-320 (FUEL ISO)"(w424) -> ()
      }
    }
    n106 = case shown="True" w87 {
      tunnel: w56 -> [_ w423]
      frame False {
      }
      frame True {
        n107 = local write "ABV-FU-330 (FUEL MAIN)"(w423) -> ()
      }
    }
    n108 = case shown="True" w85 {
      tunnel: w55 -> [_ w422]
      frame False {
      }
      frame True {
        n109 = local write "ABV-FU-340 (FUEL PURGE)"(w422) -> ()
      }
    }
    n110 = call "OX v1.2.vi"("INDICATOR INPUT"=w16, "DATA INPUT"=w15) -> ()  [unwired: 1 in, 1 out]
    "OX VENT CYCLE BUTTON LED" <- "CYCLE OX VENT BUTTON"
    "FUEL VENT CYCLE BUTTON LED" <- "CYCLE FUEL VENT BUTTON"
    "NANNY PAN LED" <- "NANNY MODE BUTTON"
    "IGN INSERTED PANEL LED" <- "IGNITOR IN BUTTON"
    "CAM GNG BUTTON LED" <- "CAM GNG BUTTON"
    "OFFICE GNG BUTTON LED" <- "OFFICE GNG BUTTON"
    "REC DATA BUTTON LED" <- "RECORD DATA BUTTON"
    "IGN INSERTED BUTTON LED" <- "IGNITOR IN BUTTON"
    "PH IND 1" <- "PH CHECK 1"
    "PH IND 2" <- "PH CHECK 2"
    "PH IND 3" <- "PH CHECK 3"
    "PH IND 4" <- "PH CHECK 4"
    "PH IND 5" <- "PH CHECK 5"
    "PH LED 1" <- "PH CHECK 1"
    "PH LED 2" <- "PH CHECK 2"
    "PH LED 3" <- "PH CHECK 3"
    "PH LED 4" <- "PH CHECK 4"
    "PH LED 5" <- "PH CHECK 5"
    "PH LED 6" <- "PH CHECK 6"
    "PH IND 6" <- "PH CHECK 6"
  }
  "Array - Numeric" <- w1
  n111 = property on="REG PRESS FU METER" class="Knob (strict)"("Scale.MarkerVals[]"=cluster{dbl, u32}[] [{0.0, 16777224}, {700.0, 16777224}, {800.0, 51245}, {900.0, 51245}, {1600.0, 16711680}, {1200.0, 16711680}, {1200.0, 13109504}, {0.0, 0}, {900.0, 16711680}, {1200.0, 16711680}] ("Scale.Marker Values[]")) -> ()  [unwired: 2 in, 2 out]
